vi "subCurveFitting.vi"(0 "signals":waveform(dbl)[](array[waveform]) caption="Signale", 1 "model description":T1 caption="Modellbeschreibung", 2 "Initial Guess Coefficient":dbl[](array[numeric]) caption="Anfänglich geschätzte Koeffizienten" format="%.2f", 5 "locations":waveform(dbl)[](array[waveform]) caption="Positionen", 7 "model":T2(ring) caption="Modell", 9 "polynomial order":i32 caption="Polynomordnung" format="%0.2f", 11 "error in":errorcluster caption="Fehler (Eingang)", 12 "linear models":string[](array[string]) caption="Lineare Modelle", 14 "max iteration":i32=200 caption="max. Iterationen") -> (4 "best fit":waveform(dbl)[](array[waveform]) caption="Beste Anpassung", 6 "residual":waveform(dbl)[](array[waveform]) caption="Rest", 8 "best fit coefficients":waveform(dbl)[](array[waveform]) caption="Koeffizienten für beste Anpassung", 10 "mse":waveform(dbl)[](array[waveform]) caption="MSE", 15 "error out":errorcluster caption="Fehler (Ausgang)")   [LabVIEW 2009]
uses:
  <vilib>/Waveform/WDTOps.llb/WDT Get Waveform Time Array DBL.vi
  <vilib>/Analysis/NI_AALPro.lvlib
  <vilib>/gmath/NI_Gmath.lvlib
panel:
  in  "Name Modifier 4":string="Rest" caption="Namen-Modifizierer 4"
  in  "Name Modifier 3":string="MSE" caption="Namen-Modifizierer 3"
  in  "Name Modifier 2":string="Koeffizienten für beste Anpassung" caption="Namen-Modifizierer 2"
  in  "Name Modifier":string="Beste Anpassung" caption="Namen-Modifizierer"
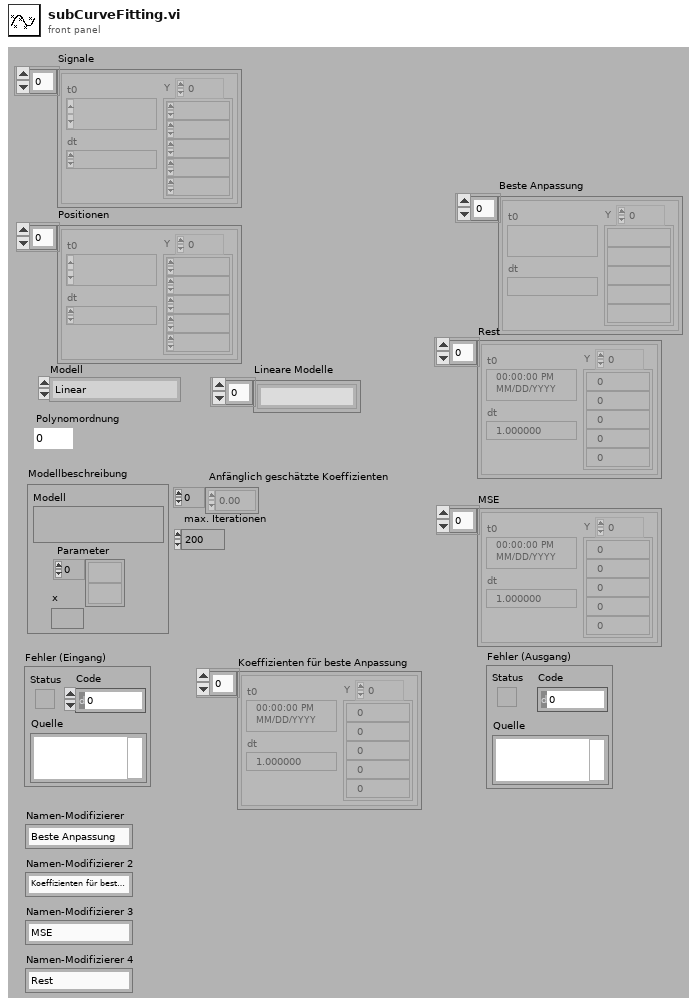
[diagram p1: front panel]
types:
  T1 = cluster{"model":string, "Parameters":string[], "x":string}
  T2 = enum16{"Linear", "Quadratic", "Cubic Spline", "Polynomial", "General LS Linear", "Non-Linear"}
  T3 = enum32{"SVD", "Givens", "Givens2", "Householder", "LU Decomposition", "Cholesky"}
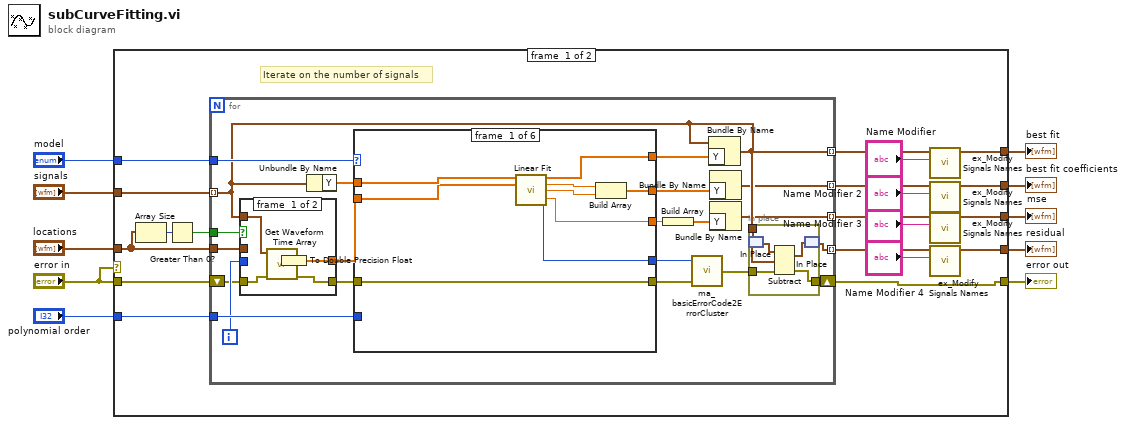
[diagram p0: block diagram]
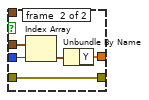
[diagram p2: hidden frame]
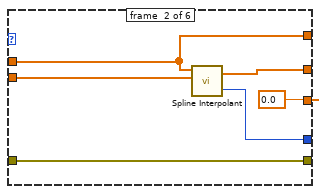
[diagram p3: hidden frame]
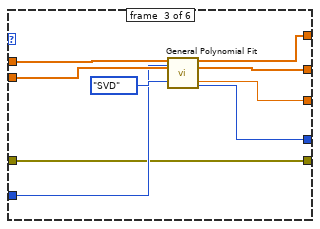
[diagram p4: hidden frame]
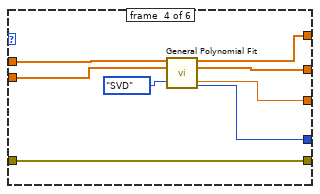
[diagram p5: hidden frame]
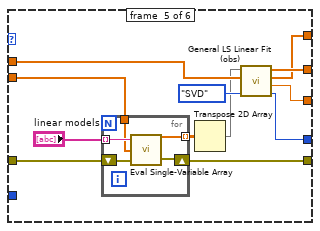
[diagram p6: hidden frame]
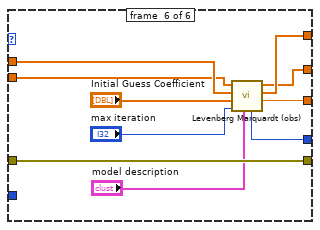
[diagram p7: hidden frame]
diagram:
  n1 = case shown="No Error" "error in" {
    tunnel: "model" -> [w30 _]
    tunnel: "error in" -> [w29 w127]
    tunnel: "polynomial order" -> [w28 _]
    tunnel: "signals" -> [w27 _]
    tunnel: "locations" -> [w25 _]
    tunnel: [w11 w127] -> w6
    tunnel: [w19 _] -> w5
    tunnel: [w18 _] -> w4
    tunnel: [w17 _] -> w3
    tunnel: [w16 _] -> w2
    frame #0 {
      # "Iterate on the number of signals"
      n2 = Array Size(array=w25) -> (size(s)=w26:i32)
      n3 = Greater Than 0?(x=w26) -> (x > 0?=w24:bool)
      n4 = for {
        tunnel: w30 -> [w50]
        tunnel: w27 -> [w39] mode=indexing
        shift-right: [w45] -> w11
        shift-left: w29 -> [w37]
        tunnel: w28 -> [w51]
        tunnel: [w44] -> w20 mode=indexing
        tunnel: [w43] -> w23 mode=indexing
        tunnel: w25 -> [w41]
        tunnel: w24 -> [w42]
        tunnel: [w34] -> w22 mode=indexing
        tunnel: [w31] -> w21 mode=indexing
        i -> [w40]
        n5 = case shown="True" w42 {
          tunnel: w41 -> [_ w67]
          tunnel: w40 -> [_ w66]
          tunnel: [w61 w64] -> w36
          tunnel: w39 -> [w62 _]
          tunnel: w37 -> [w60 w63]
          tunnel: [w59 w63] -> w38
          frame #0 {
            n6 = call-poly <vilib>:"Get Waveform Time Array.vi"("error in (no error)"=w60, "waveform in"=w62) -> ("error out"=w59:errorcluster, "X array"=w58:timestamp[])  [unwired: 8 in]
            n7 = To Double Precision Float(number=w58) -> (double precision float=w61:dbl[])
          }
          frame #1 {
            n8 = Index Array(array=w67, index=w66) -> (element=w65:waveform(dbl))
            n9 = Unbundle By Name(w65) -> ("Y"=w64:dbl[])
          }
        }
        n10 = Unbundle By Name(w39) -> ("Y"=w49:dbl[])
        n11 = case shown="\"General LS Linear\"" w50 {
          tunnel: w49 -> [w76 w80 w91 w99 w107 w123]
          tunnel: w36 -> [w75 w82 w90 w98 w105 w122]
          tunnel: [w74 w80 w88 w96 w109 w125] -> w48
          tunnel: [w71 w79 w86 w94 w110 w124] -> w35
          tunnel: [w73 w81 w89 w97 w111 w121] -> w47
          tunnel: w51 -> [_ _ w84 _ _ _]
          tunnel: [w69 0.0 ("mse") w85 w93 w108 w126] -> w33
          tunnel: w38 -> [w68 w77 w83 w92 w103 w120]
          tunnel: [w68 w77 w83 w92 w102 w120] -> w46
          frame #0 {
            n12 = call <vilib>:"Linear Fit.vi"("Y"=w76, "X"=w75) -> ("Best Linear Fit"=w74:dbl[], "slope"=w72:dbl, "intercept"=w70:dbl, "residue"=w69:dbl, "error"=w73:i32)  [unwired: 9 in]
            n13 = Build Array(w72, w70) -> (w71:dbl[])
          }
          frame #1 {
            n14 = call "Spline Interpolant.vi"("X"=w82, "Y"=w80) -> ("error"=w81:i32, "Interpolant"=w79:dbl[])  [unwired: 2 in]
          }
          frame #2 {
            n15 = call <vilib>:"General Polynomial Fit.vi"("Y"=w91, "polynomial order"=w84, "X"=w90, "algorithm"=T3."SVD") -> ("Best Polynomial Fit"=w88:dbl[], "Polynomial Coefficients"=w86:dbl[], "residue"=w85:dbl, "error"=w89:i32)  [unwired: 8 in]
          }
          frame #3 {
            n16 = call <vilib>:"General Polynomial Fit.vi"("Y"=w99, "X"=w98, "algorithm"=T3."SVD") -> ("Best Polynomial Fit"=w96:dbl[], "Polynomial Coefficients"=w94:dbl[], "residue"=w93:dbl, "error"=w97:i32)  [unwired: 9 in]
          }
          frame #4 {
            n17 = for {
              tunnel: "linear models" -> [w113] mode=indexing
              tunnel: w105 -> [w112]
              shift-right: [w115] -> w102
              shift-left: w103 -> [w116]
              tunnel: [w114] -> w104 mode=indexing
              n18 = call "Eval Single-Variable Array.vi"("error in (no error)"=w116, "X Values"=w112, "formula"=w113) -> ("error out"=w115:errorcluster, "Y Values"=w114:dbl[])
            }
            n19 = Transpose 2D Array(2D array=w104) -> (transposed array=w101:dbl[][])
            n20 = call <vilib>:"General LS Linear Fit (obs).vi"("H"=w101, "Y"=w107, "algorithm"=T3."SVD") -> ("Coefficients"=w110:dbl[], "Best Fit"=w109:dbl[], "mse"=w108:dbl, "error"=w111:i32)  [unwired: 2 in, 1 out]
          }
          frame #5 {
            n21 = call <vilib>:"Levenberg Marquardt (obs).vi"("model description"="model description", "max iteration"="max iteration", "Initial Guess Coefficient"="Initial Guess Coefficient", "Y"=w123, "X"=w122) -> ("mse"=w126:dbl, "Best Fit"=w125:dbl[], "Best Fit Coefficients"=w124:dbl[], "error"=w121:i32)  [unwired: 1 in, 2 out]
          }
        }
        n22 = Build Array(w33) -> (w32:dbl[])
        n23 = call "ma_basicErrorCode2ErrorCluster.vi"("error in (no error)"=w46, "Error Code"=w47) -> ("error out"=w52:errorcluster)  [unwired: 1 in]
        n24 = Bundle By Name(cluster=w39, "Y"=w48) -> (w43:waveform(dbl))
        n25 = Bundle By Name("Y"=w35) -> (w34:waveform(dbl))  [unwired: 1 in]
        n26 = Bundle By Name("Y"=w32) -> (w31:waveform(dbl))  [unwired: 1 in]
        n27 = in-place {
          in-place-border: w52 -> [w57]
          in-place-border: [w56] -> w45
          in-place-border: w43 -> [w54]
          n28 = in-place-match #1(w39) -> (w53:waveform(dbl))
          n29 = Subtract(1:w54, 2:w53, 4:w57) -> (0:w55:waveform(dbl), 3:w56:errorcluster)
          n30 = in-place-match #1(w55) -> (w44:waveform(dbl))
        }
      }
      n31 = call "ex_Modify Signals Names.vi"("Name Modifier"="Name Modifier", "Array of Waveforms In"=w23) -> ("Array of Waveforms Out"=w19:waveform(dbl)[])  [unwired: 8 in, 1 out]
      n32 = call "ex_Modify Signals Names.vi"("Name Modifier"="Name Modifier 2", "Array of Waveforms In"=w22) -> ("Array of Waveforms Out"=w18:waveform(dbl)[])  [unwired: 8 in, 1 out]
      n33 = call "ex_Modify Signals Names.vi"("Name Modifier"="Name Modifier 3", "Array of Waveforms In"=w21) -> ("Array of Waveforms Out"=w17:waveform(dbl)[])  [unwired: 8 in, 1 out]
      n34 = call "ex_Modify Signals Names.vi"("Name Modifier"="Name Modifier 4", "Array of Waveforms In"=w20) -> ("Array of Waveforms Out"=w16:waveform(dbl)[])  [unwired: 8 in, 1 out]
    }
    frame #1 {
    }
  }
  "error out" <- w6
  "best fit" <- w5
  "residual" <- w2
  "best fit coefficients" <- w4
  "mse" <- w3
